vi "GetAxisValuesI (SubVI).vi"(11 "read buffer":string) -> (3 "Array":dbl[](array[numeric]))   [LabVIEW 2024]
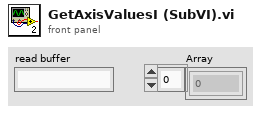
[diagram p1: front panel]
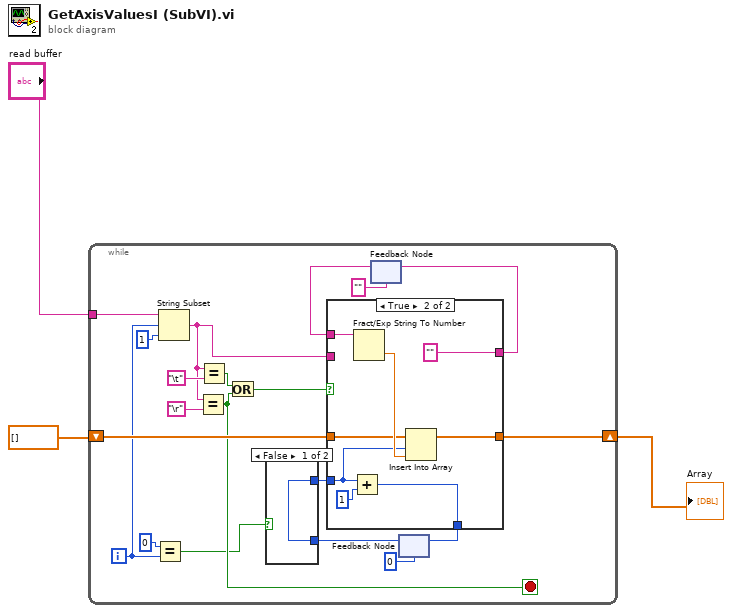
[diagram p0: block diagram]
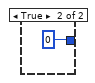
[diagram p2: hidden frame]
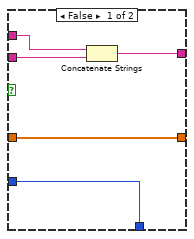
[diagram p3: hidden frame]
diagram:
  n1 = while {
    tunnel: "read buffer" -> [w22]
    shift-right: [w17] -> w3
    shift-left: dbl[] [] -> [w13]
    i -> [w9]
    stop <- w11 stop-if-true
    n2 = Equal?(x=0, y=w9) -> (x = y?=w7:bool)
    n3 = String Subset(string=w22, offset (0)=w9, length (rest)=1 ("Länge (Rest)")) -> (substring=w15:string)
    n4 = Equal?(x=w15, y="\r") -> (x = y?=w11:bool)
    n5 = Equal?(x=w15, y="\t") -> (x = y?=w14:bool)
    n6 = Or(x=w14, y=w11) -> (x .or. y?=w12:bool)
    n7 = feedback #1("") -> (w19:string)
    n8 = feedback #2(0) -> (w6:i32)
    n9 = case shown="False" w7 {
      tunnel: w6 -> [w24 _]
      tunnel: [w24 0] -> w5
      frame False {
      }
      frame True {
      }
    }
    n10 = case shown="True" w12 {
      tunnel: w5 -> [w26 w33]
      tunnel: w15 -> [w29 _]
      tunnel: w19 -> [w30 w36]
      tunnel: [w28 ""] -> w20
      tunnel: w13 -> [w27 w32]
      tunnel: [w27 w35] -> w17
      tunnel: [w26 w31] -> w4
      frame False {
        n11 = Concatenate Strings(w30, w29) -> (w28:string)
      }
      frame True {
        n12 = Add(x=w33, y=1) -> (x+y=w31:i32)
        n13 = Fract/Exp String To Number(string=w36) -> (number=w34:dbl)  [unwired: 3 in, 1 out]
        n14 = Insert Into Array(array=w32, index=w33, new element=w34) -> (w35:dbl[])
      }
    }
    n15 = feedback-in #1(w20) -> ()
    n16 = feedback-in #2(w4) -> ()
  }
  "Array" <- w3
